vi "Joysticks.vi"   [LabVIEW 2012]
uses:
  Robot Global Data.vi
  <vilib>/Rock Robotics/WPI/Joystick/WPI_JoystickGetSetRefNum.vi
types:
  T1 = typedef "WPI_JoystickDevRef.ctl" = cluster{"Device":T2}
  T2 = typedef "WPI_JoystickDeviceEnum.ctl" = enum16{"USB 1", "USB 2", "USB 3", "USB 4", "Kinect 1", "Kinect 2"}
  T3 = typedef "WPI_JoystickButtonState.ctl" = cluster{"Button 1":bool, "Button 2":bool, "Button 3":bool, "Button 4":bool, "Button 5":bool, "Button 6":bool, "Button 7":bool, "Button 8":bool, "Button 9":bool, "Button 10":bool, "Button 11":bool, "Button 12":bool}
  T4 = cluster{"axis 1 (x)":dbl, "axis 2 (y)":dbl, "axis 3 (throttle)":dbl, "axis 4":dbl, "axis 5":dbl, "axis 6":dbl}
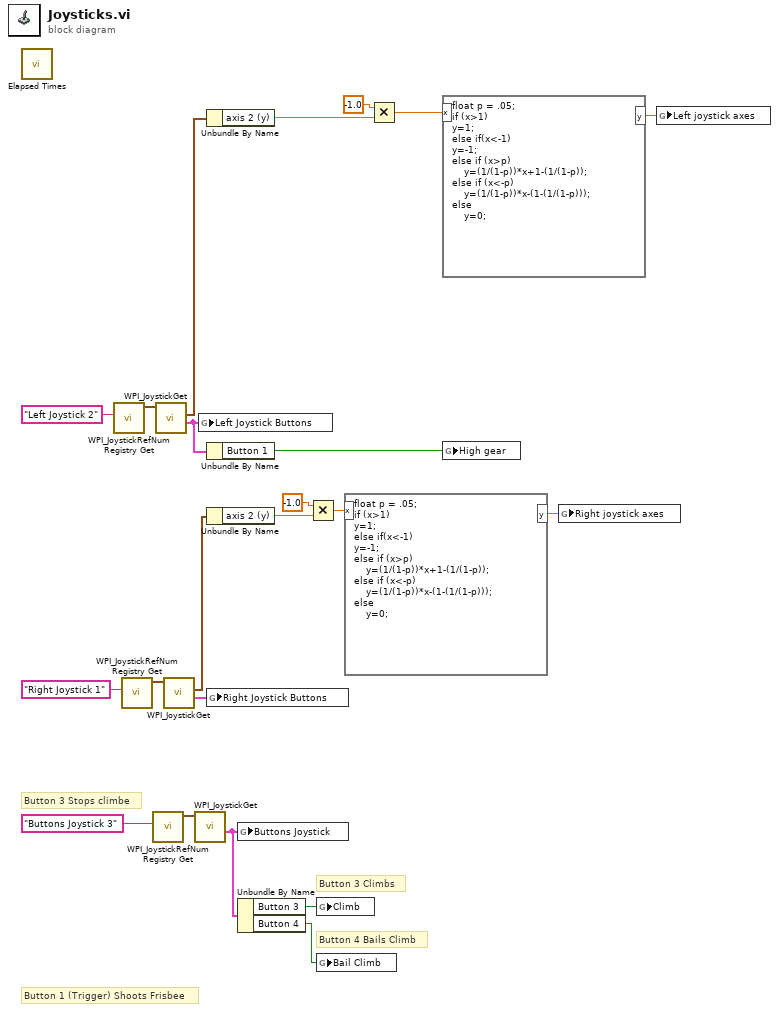
[diagram p0: block diagram]
diagram:
  # "Button 4 Bails Climb"
  # "Button 3 Climbs"
  # "Button 3 Stops climbe"
  # "Button 1 (Trigger) Shoots Frisbee"
  n1 = call "Elapsed Times.vi"() -> ()  [unwired: 3 in, 1 out]
  n2 = call <vilib>:"WPI_JoystickRefNum Registry Get.vi"("refnum name"="Left Joystick 2") -> ("JoystickDevRef"=w16:T1)  [unwired: 1 in, 9 out]
  n3 = call <vilib>:"WPI_JoystickRefNum Registry Get.vi"("refnum name"="Right Joystick 1") -> ("JoystickDevRef"=w17:T1)  [unwired: 1 in, 9 out]
  n4 = call <vilib>:"WPI_JoystickRefNum Registry Get.vi"("refnum name"="Buttons Joystick 3") -> ("JoystickDevRef"=w22:T1)  [unwired: 9 in, 1 out]
  n5 = call <vilib>:"WPI_JoystickGet.vi"("JoystickDevRef"=w16) -> ("Buttons"=w2:T3, "Axes"=w4:T4)  [unwired: 1 in, 4 out]
  n6 = call <vilib>:"WPI_JoystickGet.vi"("JoystickDevRef"=w17) -> ("Buttons"=w14:T3, "Axes"=w9:T4)  [unwired: 1 in, 4 out]
  n7 = call <vilib>:"WPI_JoystickGet.vi"("JoystickDevRef"=w22) -> ("Buttons"=w20:T3)  [unwired: 4 in, 2 out]
  n8 = global write "Robot Global Data.vi" "Left Joystick Buttons"(w2) -> ()
  n9 = Unbundle By Name(w4) -> ("axis 2 (y)"=w5:dbl)
  n10 = Unbundle By Name(w2) -> ("Button 1"=w1:bool)
  n11 = Unbundle By Name(w9) -> ("axis 2 (y)"=w10:dbl)
  n12 = global write "Robot Global Data.vi" "Right Joystick Buttons"(w14) -> ()
  n13 = global write "Robot Global Data.vi" "Buttons Joystick"(w20) -> ()
  n14 = Unbundle By Name(w20) -> ("Button 3"=w18:bool, "Button 4"=w19:bool)
  n15 = Multiply(x=-1.0, y=w10) -> (x*y=w11:dbl)
  n16 = global write "Robot Global Data.vi" "Climb"(w18) -> ()
  n17 = global write "Robot Global Data.vi" "Bail Climb"(w19) -> ()
  n18 = formula code="float p = .05; \nif (x>1)\ny=1;\nelse if(x<-1)\ny=-1;\nelse if (x>p)\n    y=(1/(1-p))*x+1-(1/(1-p));\nelse if (x<-p) \n    y=(1/(1-p))*x-(1-(1/(1-p)));\nelse\n    y=0;"("x"=w11) -> ("y"=w8:dbl)
  n19 = Multiply(x=-1.0, y=w5) -> (x*y=w6:dbl)
  n20 = formula code="float p = .05; \nif (x>1)\ny=1;\nelse if(x<-1)\ny=-1;\nelse if (x>p)\n    y=(1/(1-p))*x+1-(1/(1-p));\nelse if (x<-p) \n    y=(1/(1-p))*x-(1-(1/(1-p)));\nelse\n    y=0;"("x"=w6) -> ("y"=w3:dbl)
  n21 = global write "Robot Global Data.vi" "High gear"(w1) -> ()
  n22 = global write "Robot Global Data.vi" "Right joystick axes"(w8) -> ()
  n23 = global write "Robot Global Data.vi" "Left joystick axes"(w3) -> ()
